vi "forloop_PH.vi"() -> ()   [LabVIEW 2021]
panel:
  out "numer iteracji":dbl
  in  "liczba iteracji":dbl
  out "Liczby losowe":dbl(graph)
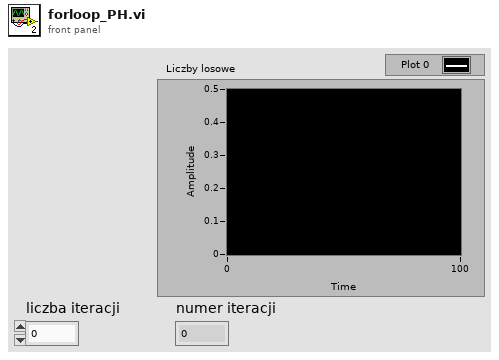
[diagram p1: front panel]
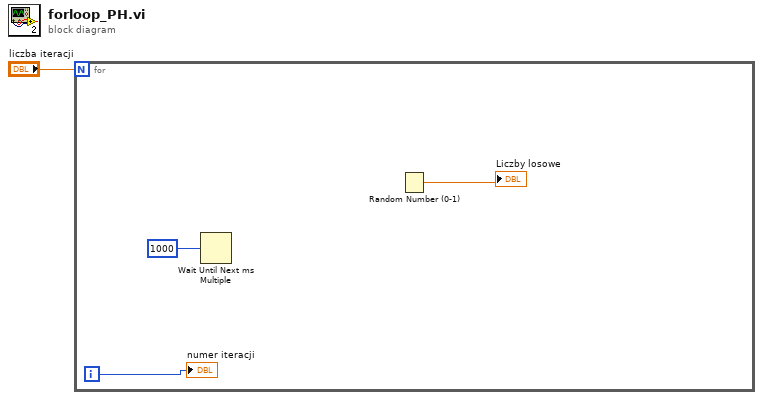
[diagram p0: block diagram]
diagram:
  n1 = for {
    N: "liczba iteracji" -> [_]
    i -> [w2]
    n2 = Wait Until Next ms Multiple(millisecond multiple=u32 1000 ("millisecond timer value")) -> ()  [unwired: 1 out]
    n3 = Random Number (0-1)() -> (number: 0 to 1=→"Liczby losowe":dbl)
    "numer iteracji" <- w2
  }
